vi "MultiRecEncoderLaser_Synchronizer.vi"(8 "error in":errorcluster, 9 "Initial?":bool, 10 "InputParams.":variant) -> (0 "error out":errorcluster, 2 "Return out":variant)   [LabVIEW 2014]
uses:
  ControlDef/QueueRefs.ctl
  ControlDef/LaserCtrl_Method.ctl
  ControlDef/States-AToF.ctl
  <instrlib>/GenericDAQ/VI/GenericDAQ_Ctrl_Queue.ctl
  <instrlib>/GenericDAQ/VI/GenericDAQ_State.ctl
  <instrlib>/ESP300/Public/Data/ESP300_State.ctl
  <instrlib>/DG535/Command/DG535_States.ctl
  Hardware/BNC(QuantumComposers)/BNC_States.ctl
  Hardware/FemtoLaser(Legacy)/Laser_Status.ctl
  Hardware/DAQmx(Legacy)/DAQmx_Status.ctl
  ControlDef/Signal.ctl
  ProcessMethods/SignalAverager/ProcessStates.ctl
  Files/WriterState.ctl
  <instrlib>/GenericDAQ/VI/GenericDAQ_Signal.ctl
  Hardware/EPM2000(Legacy)/EPM2K_Status.ctl
  Hardware/BNC(QuantumComposers)/SetSystemTypedef.ctl
  <vilib>/Utility/error.llb/Error Cluster From Error Code.vi
  <vilib>/ErrorRing/Error Ring.xnode
  <instrlib>/DG535/SRS_DG535_Lib.lvlib
  <instrlib>/GenericDAQ/GenericDAQ.lvlib
  <instrlib>/ESP300/ESP300.lvlib
panel:
  out "Segment#":i32
  out "Wait cts BNC":i32
  out "stage return":string
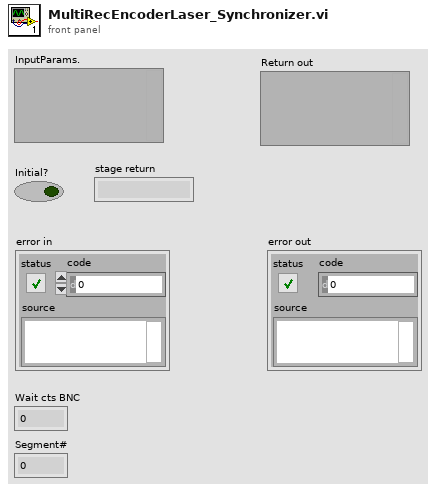
[diagram p1: front panel]
types:
  T1 = typedef "QueueRefs.ctl" = cluster{"LaserCtrlMethod":T2, "Apps":refnum<queue>, "MainDAQCoreQueue":refnum<queue>, "Micos":refnum<queue>, "ESP300":refnum<queue>, "SMC100":refnum<queue>, "SRS DG535":refnum<queue>, "BNC":refnum<queue>, "SDG_ii":refnum<queue>, "NI-USB_DAQmx":refnum<queue>, "ProcCore_CtrlQueue":refnum<queue>, "WriterCtrl":refnum<queue>, "WriterSIG":refnum<queue>, "Feedback":refnum<queue>, "EPM2000":refnum<queue>, "InfoRef":refnum<vi>, "AppsLock":T3, "ProcCore_SignalBuffer":refnum<queue>}
  T2 = typedef "LaserCtrl_Method.ctl" = enum16{"SRS_DG535", "BNC", "SDG_II", "GenericDAQ_Sim"}
  T3 = typedef "Semaphore RefNum" = refnum<k1>
  T4 = typedef "ESP300.lvlib/ESP300_State.ctl" = cluster{"State":enum16{"Initialize", "SetDefaultConfig", "Close", "Quit", "Identify", "MoveAbs", "MoveAbs_all", "MoveRel", "MoveRel_all", "STOP", "Origin/Home", "WaitStop", "QueryStatus", "UpdateXPos", "UpdateAll", "SetVelocity", "SetAcceleration", "ClearErr", "LogMessage", "MotorEnable(1)", "EnableAxis", "JoyStick", "GetVelocity", "GetAcceleration", "SendCmd", "SetSoftLimits", "Beep", "_SettingReturn", "SoftReset"}, "Params.":variant}
  T5 = typedef "BNC_States.ctl" = cluster{"State":enum16{"Initialize", "Set System", "Set C-Input", "Set C-Mode", "Set C-Output", "Set C-Enable", "Manl_Trig", "Run", "Stop", "Query C Number", "Query Status", "Close", "Quit"}, "Para.":variant}
  T6 = enum16{"Disabled", "Triggered", "Gated", "Triggered & Gated"}
  T7 = enum16{"Normal", "Single Shot", "Duty Cycle", "Burst"}
  T8 = typedef "SetSystemTypedef.ctl" = cluster{"Mode":enum16{"Normal", "Single Shot", "Duty Cycle", "Burst"}, "Sys Ext Mode":enum16{"Disabled", "Triggered", "Gated", "Triggered & Gated"}, "Rep.Rate":dbl, "Burst#":i32}
  T9 = enum16{"Normal", "Continuous", "MultiRecord", "HwAverage"}
  T10 = typedef "GenericDAQ.lvlib/GenericDAQ_Ctrl_Queue.ctl" = cluster{"GenericDAQ State":T11, "Variant":variant}
  T11 = typedef "GenericDAQ.lvlib/GenericDAQ_State.ctl" = enum16{"Enumerate", "Open", "Close", "CloseAll", "Reset", "Quit", "==Settings==", "SetAcquisition_", "SetChannels_", "SetTrigger_", "SetAnalogTrigDetector_", "SetSegment#_", "SetAll_AcquChTrig_", "fConfigurate", "fStart", "GetStatus", "_WaitForDone/Idle", "_GetData", "GetAcquisition", "GetChannels", "GetTrigger", "GetAll_AcquChTrig", "Abort", "==Messaging==", "_PushDataOut", "GetStat_", "GetConfig_", "==ModeSetup==", "SetSignalBuffer_", "SetMode_", "SetSecondaryDataRef._", "SetDynamicBuffer_", "==AnalogOut==", "GetChannelCount_AO", "fStart_AO", "SetChEnable_AO", "SetConfig_AO", "SetFuncData_AO", "SetOffset_AO_", "SetMasterNode_AO", "SetStates_AO", "SetSymetry_AO", "SetTriggerSource_AO", "==Trigger==", "ManualTrigger", "===Sync===", "LineStart", "LineEnd", "FrameStart", "FrameEnd", "EOL_PassThrough", "SOL_PassThrough"}
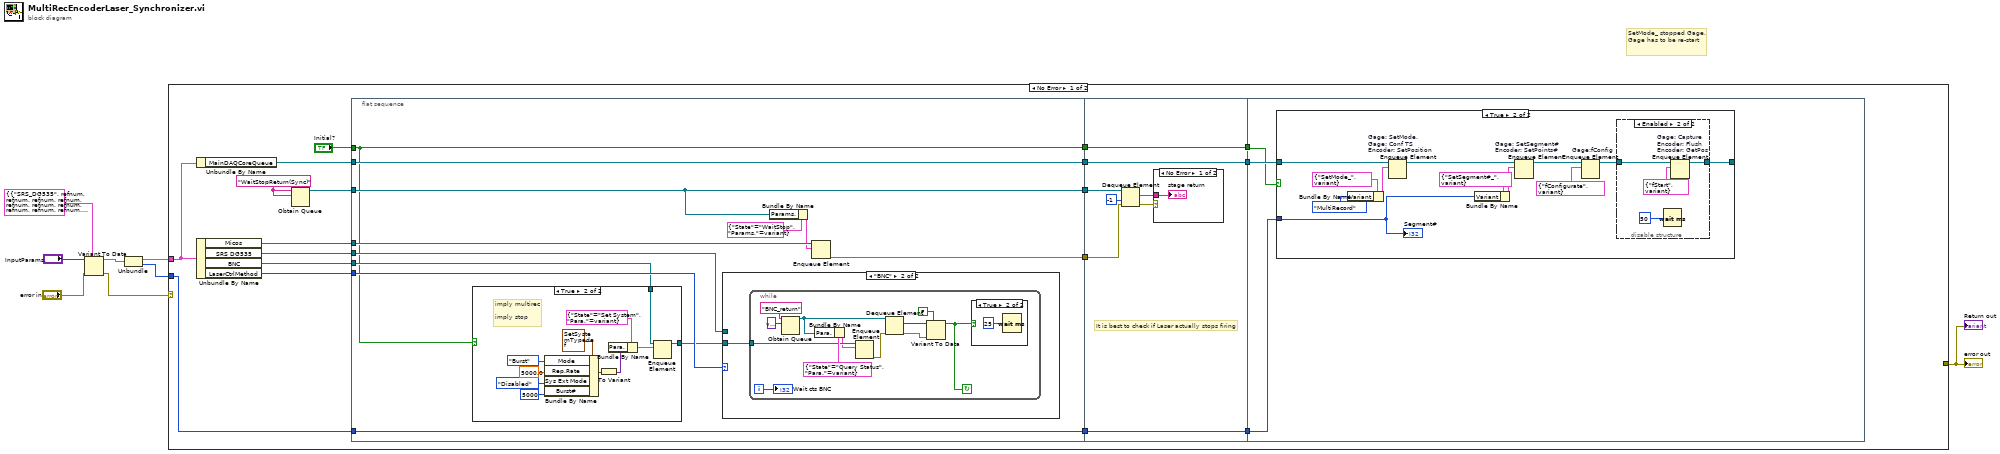
[diagram p0: block diagram]
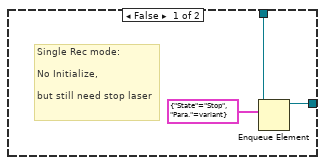
[diagram p2: hidden frame]
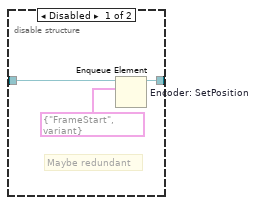
[diagram p7: hidden frame]
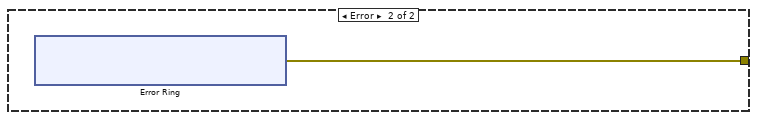
[diagram p8: hidden frame]
diagram:
  # "SetMode_ stopped Gage,\nGage has to be re-start"
  n1 = Variant To Data(error in="error in", type=cluster{"Queue cluster":T1, "Segment#":i32} {"Queue cluster"={"LaserCtrlMethod"=enum."SRS_DG535", "Apps"=refnum, "MainDAQCoreQueue"=refnum, "Micos"=refnum, "ESP300"=refnum, "SMC100"=refnum, "SRS DG535"=refnum, "BNC"=refnum, "SDG_ii"=refnum, "NI-USB_DAQmx"=refnum, "ProcCore_CtrlQueue"=refnum, "WriterCtrl"=refnum, "WriterSIG"=refnum, "Feedback"=refnum, "EPM2000"=refnum, "InfoRef"=refnum, "AppsLock"=refnum, "ProcCore_SignalBuffer"=refnum}, "Segment#"=0}, Variant="InputParams.") -> (data=w6:cluster{"Queue cluster":T1, "Segment#":i32}, error out=w3:errorcluster)
  n2 = Unbundle(w6) -> ("Queue cluster"=w5:T1, "Segment#"=w2:i32)
  n3 = case shown="No Error" w3 {
    tunnel: w5 -> [w17 _]
    tunnel: w2 -> [w14 _]
    tunnel: [_ w99] -> w1
    frame No Error {
      w12 = "WaitStopReturn(Sync)" ("name (unnamed)")
      n4 = Unbundle By Name(w17) -> ("MainDAQCoreQueue"=w18:refnum<queue>)
      n5 = Unbundle By Name(w17) -> ("Micos"=w20:refnum<queue>, "SRS DG535"=w21:refnum<queue>, "BNC"=w23:refnum<queue>, "LaserCtrlMethod"=w22:T2)
      n6 = Obtain Queue(name (unnamed)=w12, element data type=w12) -> (queue out=w19:refnum<queue>)  [unwired: 3 in, 2 out]
      n7 = flat-sequence {
        tunnel: w23 -> [w29]
        tunnel: w22 -> [w38]
        tunnel: w21 -> [w37]
        tunnel: w20 -> [w36]
        tunnel: w19 -> [w31]
        tunnel: [w35] -> w26
        tunnel: w18 -> [w34]
        tunnel: [w34] -> w25
        tunnel: [w28] -> w15
        tunnel: w14 -> [w28]
        tunnel: [w31] -> w13
        tunnel: [w27] -> w10
        tunnel: "Initial?" -> [w27]
        tunnel: w26 -> [w70]
        tunnel: [w74] -> w24
        tunnel: w25 -> [w74]
        tunnel: [w73] -> w16
        tunnel: w15 -> [w73]
        tunnel: w13 -> [w72]
        tunnel: [w67] -> w11
        tunnel: w10 -> [w67]
        tunnel: w24 -> [w78]
        tunnel: w16 -> [w77]
        tunnel: w11 -> [w76]
        frame #0 {
          n8 = case shown="True" w27 {
            tunnel: [w40 w52] -> w30
            tunnel: w29 -> [w41 w51]
            frame False {
              # "Single Rec mode:\n\nNo Initialize,\n\nbut still need stop laser"
              n9 = Enqueue Element(queue=w41, element=T5 {"State"=enum."Stop", "Para."=variant}) -> (queue out=w40:refnum<queue>)  [unwired: 2 in, 2 out]
            }
            frame True {
              # "imply multirec\n\nimply stop"
              n10 = Bundle By Name(cluster=T8 {"Mode"=enum."Normal", "Sys Ext Mode"=enum."Triggered", "Rep.Rate"=0.0, "Burst#"=1}, "Mode"=T7."Burst", "Rep.Rate"=5000.0, "Sys Ext Mode"=T6."Disabled", "Burst#"=5000 ("Rep.Rate")) -> (w45:T8)
              n11 = To Variant(anything=w45) -> (Variant=w46:variant)
              n12 = Bundle By Name(cluster=T5 {"State"=enum."Set System", "Para."=variant} ("element"), "Para."=w46) -> (w42:T5)
              n13 = Enqueue Element(queue=w51, element=w42) -> (queue out=w52:refnum<queue>)  [unwired: 2 in, 2 out]
            }
          }
          n14 = case shown="\"BNC\"" w38 {
            tunnel: w30 -> [_ w53]
            tunnel: w37 -> [_ _]
            frame Default {
            }
            frame "BNC" {
              n15 = while {
                tunnel: w53 -> [w64]
                i -> [w55]
                stop <- w54 continue-if-true
                n16 = Obtain Queue(name (unnamed)="BNC_return", element data type=variant) -> (queue out=w60:refnum<queue>)  [unwired: 3 in, 2 out]
                n17 = Bundle By Name(cluster=T5 {"State"=enum."Query Status", "Para."=variant} ("element"), "Para."=w60) -> (w63:T5)
                n18 = Enqueue Element(queue=w64, element=w63) -> (error out=w59:errorcluster)  [unwired: 2 in, 2 out]
                n19 = Dequeue Element(queue=w60, error in (no error)=w59) -> (element=w58:variant, error out=w56:errorcluster)  [unwired: 1 in, 2 out]
                n20 = Variant To Data(error in=w56, type=FALSE, Variant=w58) -> (data=w54:bool)  [unwired: 1 out]
                n21 = case shown="True" w54 {
                  frame False {
                  }
                  frame True {
                    n22 = Wait (ms)(milliseconds to wait=u32 25) -> ()  [unwired: 1 out]
                  }
                }
                "Wait cts BNC" <- w55
              }
            }
          }
          n23 = Bundle By Name(cluster=T4 {"State"=enum."WaitStop", "Params."=variant} ("element"), "Params."=w31) -> (w32:T4)
          n24 = Enqueue Element(queue=w36, element=w32) -> (error out=w35:errorcluster)  [unwired: 2 in, 2 out]
        }
        frame #1 {
          # "It is best to check if Laser actually stops firing"
          n25 = Dequeue Element(queue=w72, timeout in ms (-1)=-1, error in (no error)=w70) -> (element=w69:string, error out=w71:errorcluster)  [unwired: 2 out]
          n26 = case shown="No Error" w71 {
            tunnel: w69 -> [w75 _]
            frame No Error {
              "stage return" <- w75
            }
            frame Error {
            }
          }
        }
        frame #2 {
          n27 = case shown="True" w76 {
            tunnel: w78 -> [w79 w82]
            tunnel: [w79 w91] -> _
            tunnel: w77 -> [_ w88]
            frame False {
            }
            frame True {
              n28 = Bundle By Name(cluster=T10 {"GenericDAQ State"=enum."SetMode_", "Variant"=variant} ("element"), "Variant"=T9."MultiRecord" ("Mode(Gage)")) -> (w84:T10)
              n29 = Enqueue Element "Gage: SetMode,\nGage: Conf TS\nEncoder: SetPosition"(queue=w82, element=w84) -> (queue out=w81:refnum<queue>)  [unwired: 2 in, 2 out]
              n30 = Bundle By Name(cluster=T10 {"GenericDAQ State"=enum."SetSegment#_", "Variant"=variant} ("element"), "Variant"=w88) -> (w90:T10)
              n31 = Enqueue Element "Gage: SetSegment#\nEncoder: SetPoints#"(queue=w81, element=w90) -> (queue out=w80:refnum<queue>)  [unwired: 2 in, 2 out]
              n32 = Enqueue Element "Gage:fConfig"(queue=w80, element=T10 {"GenericDAQ State"=enum."fConfigurate", "Variant"=variant}) -> (queue out=w86:refnum<queue>)  [unwired: 2 in, 2 out]
              n33 = disable-structure shown="Enabled" {
                disable-tunnel: w86 -> [w93 w97]
                disable-tunnel: [w92 w96] -> w91
                frame Disabled {
                  # "Maybe redundant"
                  n34 = Enqueue Element "Encoder: SetPosition"(queue=w93, element=T10 {"GenericDAQ State"=enum."FrameStart", "Variant"=variant}) -> (queue out=w92:refnum<queue>)  [unwired: 2 in, 2 out]
                }
                frame Enabled {
                  n35 = Wait (ms)(milliseconds to wait=u32 50) -> ()  [unwired: 1 out]
                  n36 = Enqueue Element "Gage: Capture\nEncoder: Flush\nEncoder: GetPos"(queue=w97, element=T10 {"GenericDAQ State"=enum."fStart", "Variant"=variant}) -> (queue out=w96:refnum<queue>)  [unwired: 2 in, 2 out]
                }
              }
              "Segment#" <- w88
            }
          }
        }
      }
    }
    frame Error {
      n37 = xnode "Error Ring"() -> ("error out"=w99:errorcluster)
    }
  }
  "Return out" <- w1
  "error out" <- w1
